vi "Monitor Current Step.vi"(0 "VISA resource name":refnum<visa-resource-name>, 1 "Unit Address (1)":i16=1, 5 "Status To Read (0: Current Profile File)":u16(ring) items=["Current Profile File Number", "Current Profile Step Number", "Current Profile Step Type", "Profile Ramp Waiting", "Profile Waiting For Event 1", "Profile Waiting For Event 2", "Profile Waiting For Event 3", "Profile Waiting For Event 4", "Profile Waiting Analog Input 1", "Profile Waiting Analog Input 2", "Profile Waiting Analog Input 3", "Digital Output 1", "Digital Output 2", "Digital Output 3", "Digital Output 4", "Digital Output 5", "Digital Output 6", "Digital Output 7", "Digital Output 8", "Hours Remaining", "Minutes Remaining", "Seconds Remaining", "Set Point Ch1", "Set Point Ch2", "Ch1 PID Set", "Ch2 PID Set", "Last Jump Count", "Last Jump File", "Jump Step", "End Setpoint Ch1", "End Setpoint Ch2"], 11 "error in (no error)":errorcluster {"code" format="%.0x"}) -> (4 "VISA resource name out":refnum<visa-resource-name>, 6 "Value":dbl format="%.2f", 15 "error out":errorcluster {"code" format="%.0x"})   [LabVIEW 2010]
doc: "This VI monitors current step, while profile is running."
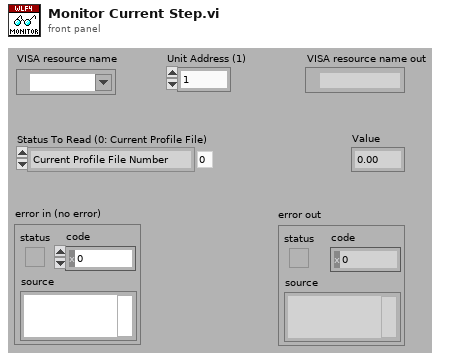
[diagram p1: front panel]
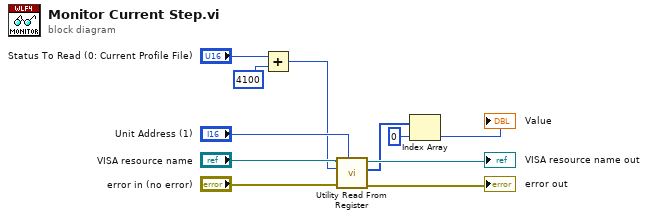
[diagram p0: block diagram]
diagram:
  n1 = Add(x="Status To Read (0: Current Profile File)", y=u16 4100) -> (x+y=w4:u16)
  n2 = call "Utility Read From Register.vi"("Unit Address (1)"="Unit Address (1)", "error in (no error)"="error in (no error)", "Register Address (0)"=w4, "VISA resource name"="VISA resource name") -> ("error out"=→"error out":errorcluster, "Data"=w2:i16[], "VISA resource name out"=→"VISA resource name out":refnum<visa-resource-name>)  [unwired: 5 in]
  n3 = Index Array(array=w2, index=0) -> (element=→"Value":i16)
